vi "Add Timer.vi"(10 "Timer":refnum<class "Timer.lvclass">, 11 "UserEventTimer in":refnum<class "TimerEngine.lvclass">) -> (3 "UserEventTimer out":refnum<class "TimerEngine.lvclass">)   [LabVIEW 2017, in "TimerEngine.lvlib" / "TimerEngine.lvclass"]
uses:
  TimerEngine.lvclass
  _TimerClass/Timer.lvclass
  TimerEngine.lvclass/TimerEngine.ctl
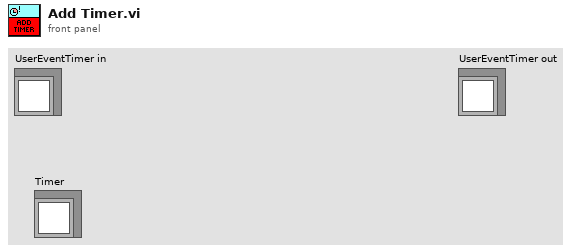
[diagram p1: front panel]
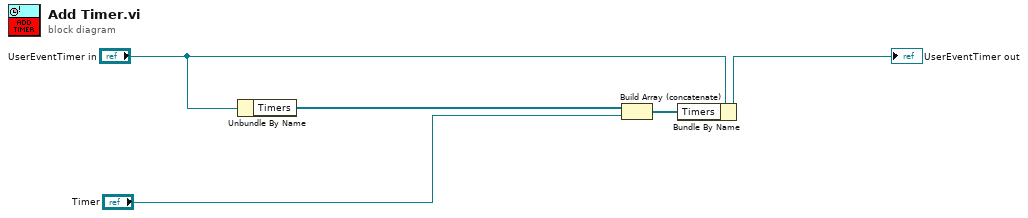
[diagram p0: block diagram]
diagram:
  n1 = Unbundle By Name("UserEventTimer in") -> ("Timers"=w3:refnum<class "Timer.lvclass">[])
  n2 = Build Array (concatenate)(w3, "Timer") -> (w2:refnum<class "Timer.lvclass">[])
  n3 = Bundle By Name(cluster="UserEventTimer in", "Timers"=w2) -> (→"UserEventTimer out":refnum<class "TimerEngine.lvclass">)
